vi "CONEX-ALL Set Identifier v2.vi"(9 "Stage Identifier":string, 11 "Connection Cluster in":T1) -> (3 "Connection Cluster out":T1)   [LabVIEW 2013]
doc: "ID - Set Identifier\n\nIdentifier is for attached device. (e.g. optical sensor, motion stage, etc.)\n\nInput: New Identifier"
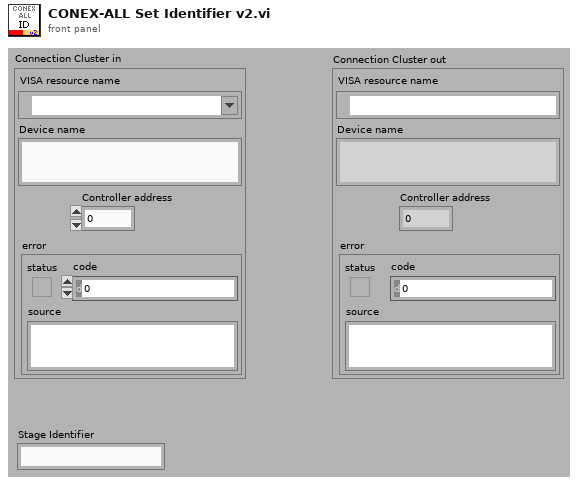
[diagram p1: front panel]
types:
  T1 = cluster{"VISA resource name":refnum<visa-resource-name>, "Device name":string, "Controller address":i32, "error":errorcluster}
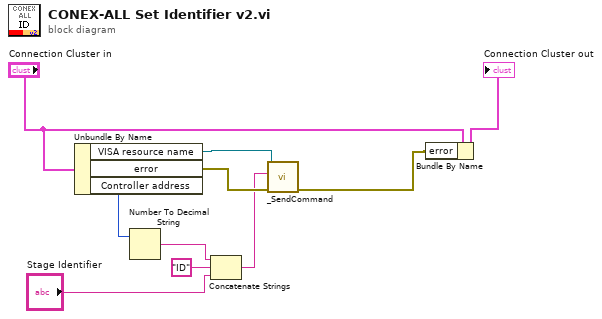
[diagram p0: block diagram]
diagram:
  n1 = Unbundle By Name("Connection Cluster in") -> ("VISA resource name"=w7:refnum<visa-resource-name>, "error"=w5:errorcluster, "Controller address"=w1:i32)
  n2 = Number To Decimal String(number=w1) -> (decimal integer string=w10:string)  [unwired: 1 out]
  n3 = Concatenate Strings(w10, "ID" ("strCommand"), "Stage Identifier") -> (w2:string)
  n4 = call "_SendCommand.vi"("error in"=w5, "Command"=w2, "Instrument Channel"=w7) -> ("error out"=w6:errorcluster)  [unwired: 7 in, 1 out]
  n5 = Bundle By Name(cluster="Connection Cluster in", "error"=w6) -> (→"Connection Cluster out":T1)
